vi "FindNameInTree.vi"(8 "error in (no error)":errorcluster, 10 "Event Registration Refnum":refnum<event-registration>, 11 "TreeReference":refnum<vi>) -> (0 "error out":errorcluster)   [LabVIEW 2013, in "FindName Task_Manager.lvlib"]
doc: "Provides a mechanism to allow the user to specify a string to be searched for. Tree items containing a match are highlighted. Also, a count of matching tree items is displayed, along with a count of all tree items."
uses:
  FindName Task_Manager.lvlib
  <vilib>/Utility/miscctls.llb/LVSelectionTypeDef.ctl
  <vilib>/Utility/error.llb/DialogType.ctl
panel:
  in  "Close":bool
  out "Found/Total =":string
  in  "NameToFind":string caption="Find ="
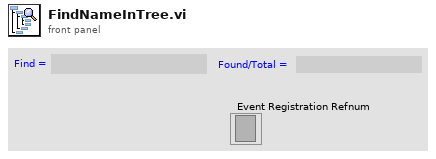
[diagram p1: front panel]
types:
  T1 = typedef "LVSelectionTypeDef.ctl" = cluster{"Selection Start":u32, "Selection End":u32}
  T2 = typedef "DialogType.ctl" = u16
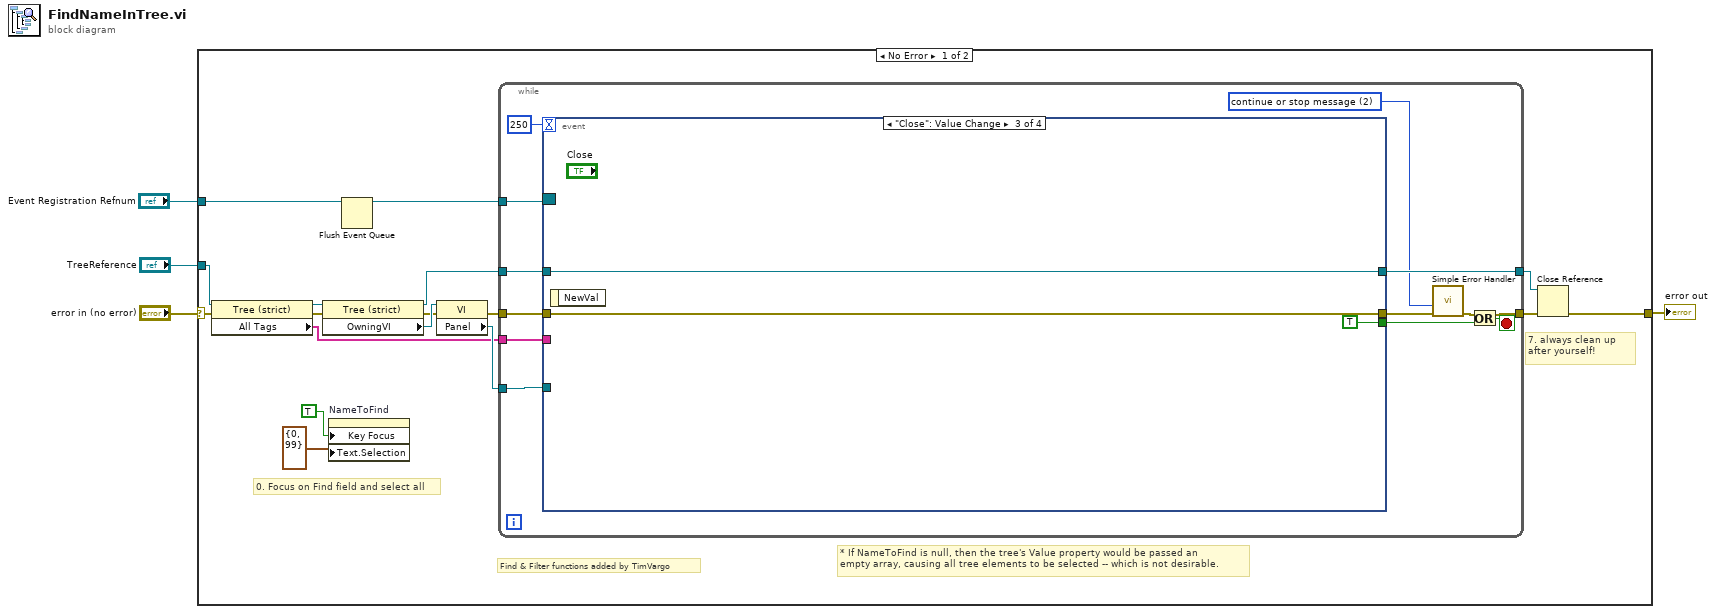
[diagram p0: block diagram]
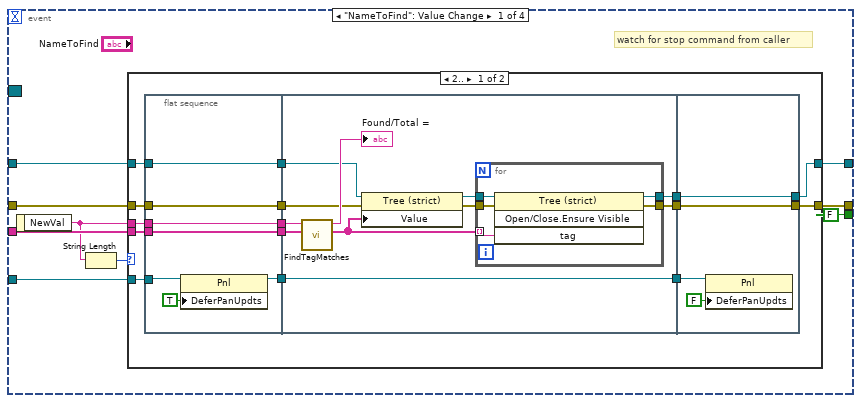
[diagram p2: hidden frame]
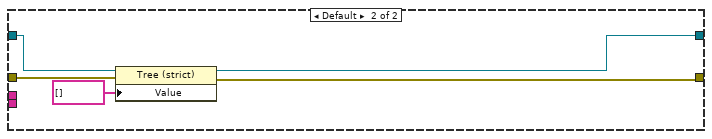
[diagram p3: hidden frame]
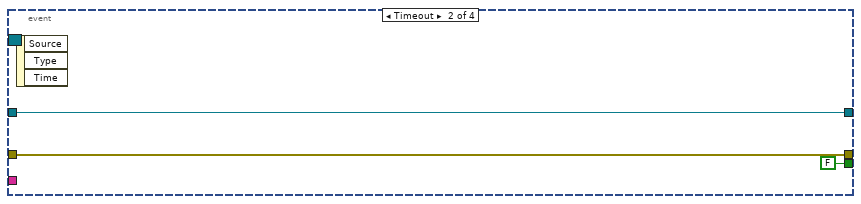
[diagram p4: hidden frame]
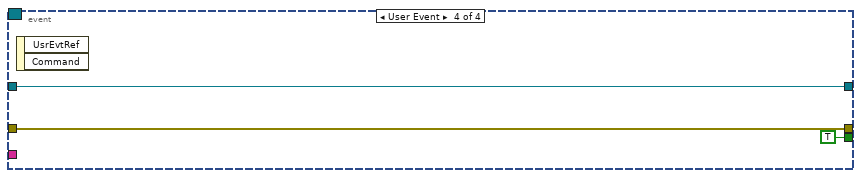
[diagram p5: hidden frame]
diagram:
  n1 = case shown="No Error" "error in (no error)" {
    selector: "error in (no error)" -> [w9 w99]
    tunnel: "TreeReference" -> [w8 _]
    tunnel: [w11 w99] -> w2
    tunnel: "Event Registration Refnum" -> [w12 _]
    frame No Error {
      # "0. Focus on Find field and select all"
      # "Find & Filter functions added by TimVargo"
      # "* If NameToFind is null, then the tree's Value property would be passed an \nempty array, causing all tree elements to be selected -- which is not desirable."
      # "7. always clean up after yourself!"
      n2 = property on="Property Node" class="Tree (strict)"(reference=w8, error in=w9) -> (reference out=w7:refnum<vi>, error out=w6:errorcluster, "All Tags"=w5:string[])
      n3 = property class="Tree (strict)"(reference=w7, error in=w6) -> (reference out=w16:refnum<vi>, error out=w18:errorcluster, "OwningVI"=w20:refnum<vi>)
      n4 = property on="NameToFind" class="Str"("Key Focus"=TRUE, "Text.Selection"=T1 {"Selection Start"=0, "Selection End"=99}) -> ()  [unwired: 2 in, 2 out]
      n5 = Flush Event Queue(0:w12) -> (8:w10:refnum<event-registration>)  [unwired: 5 in, 2 out]
      n6 = property class="VI"(reference=w20, error in=w18) -> (error out=w17:errorcluster, "Panel"=w19:refnum<vi>)  [unwired: 1 out]
      n7 = while {
        tunnel: w16 -> [w31]
        tunnel: [w33] -> w21
        tunnel: w17 -> [w30]
        tunnel: w5 -> [w29]
        tunnel: w19 -> [w28]
        tunnel: [w25] -> w15
        tunnel: w10 -> [w22]
        stop <- w23 stop-if-true
        w26 = T2 2 items=["no dialog", "OK message", "continue or stop message", "OK message + warnings", "continue/stop + warnings"] ("type of dialog (OK msg:1)")
        n8 = event shown="[2] \"Close\": Value Change" {
          selector: w22 -> [_ _ _ _]
          dyn-events: _ -> [_ _ _ _]
          timeout: 250 -> [_ _ _ _]
          tunnel: w31 -> [w41 w91 w94 w96]
          tunnel: [FALSE FALSE TRUE TRUE] -> w24
          tunnel: [w42 w91 w94 w96] -> w33
          tunnel: w30 -> [w40 w92 w93 w98]
          tunnel: w29 -> [w38 _ _ _]
          tunnel: w28 -> [w37 _ _ _]
          tunnel: [w34 w92 w93 w98] -> w27
          event "NameToFind": Value Change {
            # "watch for stop command from caller"
            n9 = event-data() -> ("NewVal"=w35:string)  [unwired: 1 in]
            n10 = String Length(string=w35) -> (length=w36:i32)
            n11 = case shown="2.." w36 {
              tunnel: [w57 w88] -> w42
              tunnel: w41 -> [w54 w89]
              tunnel: w40 -> [w55 w86]
              tunnel: w38 -> [w56 _]
              tunnel: w37 -> [w48 _]
              tunnel: w35 -> [w45 _]
              tunnel: [w44 w85] -> w34
              frame 2.. {
                n12 = flat-sequence {
                  tunnel: w54 -> [w61]
                  tunnel: w55 -> [w62]
                  tunnel: w56 -> [w63]
                  tunnel: w45 -> [w64]
                  tunnel: [w64] -> w53
                  tunnel: [w63] -> w52
                  tunnel: [w62] -> w51
                  tunnel: [w61] -> w50
                  tunnel: w48 -> [w60]
                  tunnel: [w59] -> w46
                  tunnel: w53 -> [w74]
                  tunnel: w52 -> [w70]
                  tunnel: w51 -> [w69]
                  tunnel: w50 -> [w68]
                  tunnel: [w71] -> w49
                  tunnel: [w67] -> w47
                  tunnel: w46 -> [w67]
                  tunnel: [w65] -> w43
                  tunnel: [w84] -> w57
                  tunnel: w49 -> [w84]
                  tunnel: w47 -> [w83]
                  tunnel: [w81] -> w44
                  tunnel: w43 -> [w81]
                  frame #0 {
                    n13 = property class="Pnl"(reference=w60, "DeferPanUpdts"=TRUE ("Defer Panel Updates")) -> (reference out=w59:refnum<vi>)  [unwired: 1 in, 1 out]
                  }
                  frame #1 {
                    n14 = call "FindTagMatches.vi"("All Tags"=w70, "NameToFind"=w74) -> ("Found"=w66:string[], "ResultString"=→"Found/Total =":string)  [unwired: 7 in, 1 out]
                    n15 = property class="Tree (strict)"(reference=w68, error in=w69, "Value"=w66) -> (reference out=w73:refnum<vi>, error out=w72:errorcluster)
                    n16 = for {
                      tunnel: [w80] -> w65
                      tunnel: w72 -> [w79]
                      tunnel: w73 -> [w78]
                      tunnel: [w77] -> w71
                      tunnel: w66 -> [w76] mode=indexing
                      n17 = invoke class="Tree (strict)" method="Open/Close.Ensure Visible"(reference=w78, error in=w79, "tag"=w76) -> (reference out=w77:refnum<vi>, error out=w80:errorcluster)  [unwired: 1 in, 2 out]
                    }
                  }
                  frame #2 {
                    n18 = property class="Pnl"(reference=w83, "DeferPanUpdts"=FALSE ("Defer Panel Updates")) -> ()  [unwired: 1 in, 2 out]
                  }
                }
              }
              frame Default {
                n19 = property class="Tree (strict)"(reference=w89, error in=w86, "Value"=string[] []) -> (reference out=w88:refnum<vi>, error out=w85:errorcluster)
              }
            }
          }
          event Timeout {
            n20 = event-data() -> ()  [unwired: 1 in, 3 out]
          }
          event "Close": Value Change {
            n21 = event-data() -> ()  [unwired: 1 in, 1 out]
          }
          event User Event {
            n22 = event-data() -> ()  [unwired: 1 in, 2 out]
          }
        }
        n23 = call <vilib>:"Simple Error Handler.vi"("type of dialog (OK msg:1)"=w26, "error in (no error)"=w27) -> ("error out"=w25:errorcluster)  [unwired: 3 in, 4 out]
        n24 = Or(x=w25, y=w24) -> (x .or. y?=w23:bool)
      }
      n25 = Close Reference(reference=w21, error in (no error)=w15) -> (error out=w11:errorcluster)
    }
    frame Error {
    }
  }
  "error out" <- w2
